vi "Create Menus.vi"(6 "menu options":cluster{"open":bool, "save":bool, "view":bool}={"open"=TRUE, "save"=FALSE, "view"=FALSE}, 8 "error in (no error)":errorcluster, 11 "Application Data in":T1) -> (0 "error out":errorcluster, 3 "Application Data out":T1)   [LabVIEW 2017, in "DSF Configuration Utility.lvlib"]
uses:
  DSF Configuration Utility.lvlib
  Application Data.ctl
  <vilib>/National Instruments/Data Sharing Framework Core/Data Sharing Framework Core.lvlibp/Configuration/1.0.0/Public/Controls/DSF Config Data RefNum.ctl
  View Mode.ctl
  <vilib>/National Instruments/Data Sharing Framework Core/Data Sharing Framework Core.lvlibp/Configuration/1.0.0/Data Sharing Framework Configuration.lvlib
panel:
  # "App\nData"
  # "App\nData"
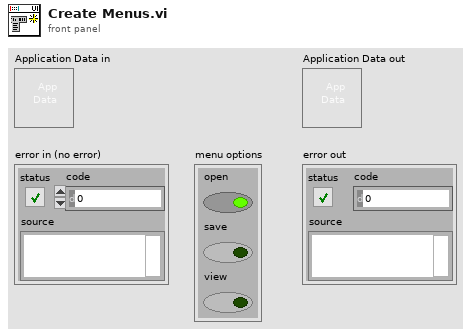
[diagram p1: front panel]
types:
  T1 = typedef "DSF Configuration Utility.lvlib/Application Data.ctl" = cluster{"Item Tree Control":refnum<vi>, "Value Tree Control":refnum<vi>, "DSF Refnum":T2, "Top-Level VI":refnum<vi>, "View State":T3, "menu reference":refnum<k9>}
  T2 = typedef "Data Sharing Framework Core.lvlibp/Data Sharing Framework Configuration.lvlib/DSF Config Data RefNum.ctl" = refnum<k1>
  T3 = typedef "DSF Configuration Utility.lvlib/View Mode.ctl" = enum16{"Tree", "List"}
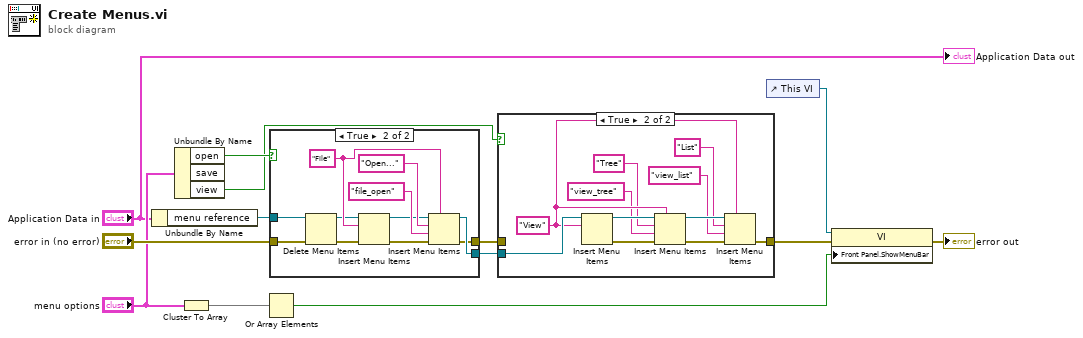
[diagram p0: block diagram]
diagram:
  n1 = Unbundle By Name("Application Data in") -> ("menu reference"=w1:refnum<k9>)
  n2 = Unbundle By Name("menu options") -> ("open"=w11:bool, "view"=w10:bool)  [unwired: 1 out]
  n3 = Cluster To Array(cluster="menu options") -> (array=w7:bool[])
  n4 = Or Array Elements(Boolean array=w7) -> (logical OR=w5:bool)
  n5 = case shown="True" w11 {
    tunnel: "error in (no error)" -> [w14 w26]
    tunnel: [w15 w24] -> w12
    tunnel: w1 -> [w15 w17]
    tunnel: [w14 w16] -> w9
    frame False {
    }
    frame True {
      w21 = "File" ("item names")
      n6 = Delete Menu Items(6:w26, 9:w17) -> (0:w25:errorcluster, 3:w18:refnum<k9>)  [unwired: 2 in]
      n7 = Insert Menu Items(6:w25, 8:w21, 9:w18) -> (0:w19:errorcluster, 3:w20:refnum<k9>)  [unwired: 3 in, 1 out]
      n8 = Insert Menu Items(5:w21, 6:w19, 7:"file_open" ("item tags"), 8:"Open..." ("item names"), 9:w20) -> (0:w16:errorcluster, 3:w24:refnum<k9>)  [unwired: 1 in, 1 out]
    }
  }
  n9 = case shown="True" w10 {
    tunnel: [w27 w38] -> w4
    tunnel: w12 -> [_ w37]
    tunnel: w9 -> [w27 _]
    frame False {
    }
    frame True {
      w35 = "View" ("item names")
      n10 = Insert Menu Items(8:w35, 9:w37) -> (0:w31:errorcluster, 3:w30:refnum<k9>)  [unwired: 4 in, 1 out]
      n11 = Insert Menu Items(5:w35, 6:w31, 7:"view_tree" ("item tags"), 8:"Tree" ("item names"), 9:w30) -> (0:w36:errorcluster, 3:w34:refnum<k9>)  [unwired: 1 in, 1 out]
      n12 = Insert Menu Items(5:w35, 6:w36, 7:"view_list" ("item tags"), 8:"List" ("item names"), 9:w34) -> (0:w38:errorcluster)  [unwired: 1 in, 2 out]
    }
  }
  n13 = control-ref of="This VI"() -> (w6:refnum<vi>)
  n14 = property class="VI"(reference=w6, error in=w4, "Front Panel.ShowMenuBar"=w5) -> (error out=→"error out":errorcluster)  [unwired: 1 out]
  "Application Data out" <- "Application Data in"
